vi "LJUD_GetNextResult.vi"(6 "GetFirst":bool=TRUE, 8 "error in":errorcluster, 11 "Handle In":i32) -> (0 "error out":errorcluster, 1 "LJE_NO_MORE_DATA_AVAILABLE":bool=TRUE, 2 "Value":dbl format="%.2f", 3 "Handle Out":i32, 5 "Channel":i32, 7 "IOType":i32)   [LabVIEW 2020]
doc: "This VI implements GetFirstResult and\nGetNextResult, which are used to step\nthrough the list of results in order.\n\nThis is a traditional technique UD\nfunction ... Add-Add-Go-Get-Get.\nSee Section 4.1 of the device's\ndatasheet for more information."
uses:
  labjackud.dll
panel:
  # "This VI implements GetFirstResult and\nGetNextResult, which are used to step\nthrough the list of results in order.\n\nThis is a traditional technique UD\nfunction ... Add-Add-Go-Get-Get.\nSee Section 4.1 of the device's\ndatasheet for more information."
  # "This VI is used for GetFirst or GetNext."
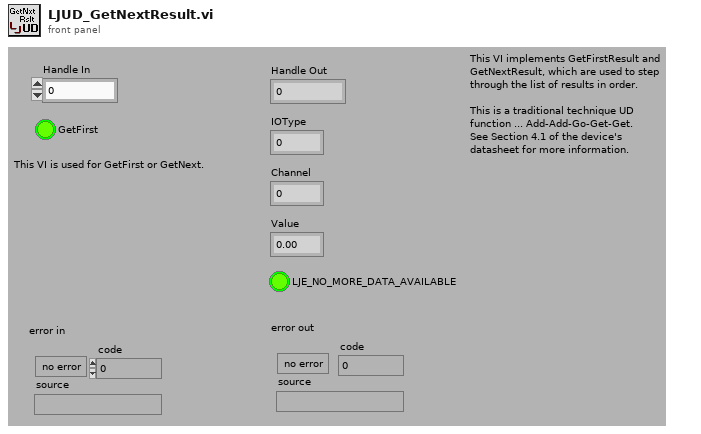
[diagram p1: front panel]
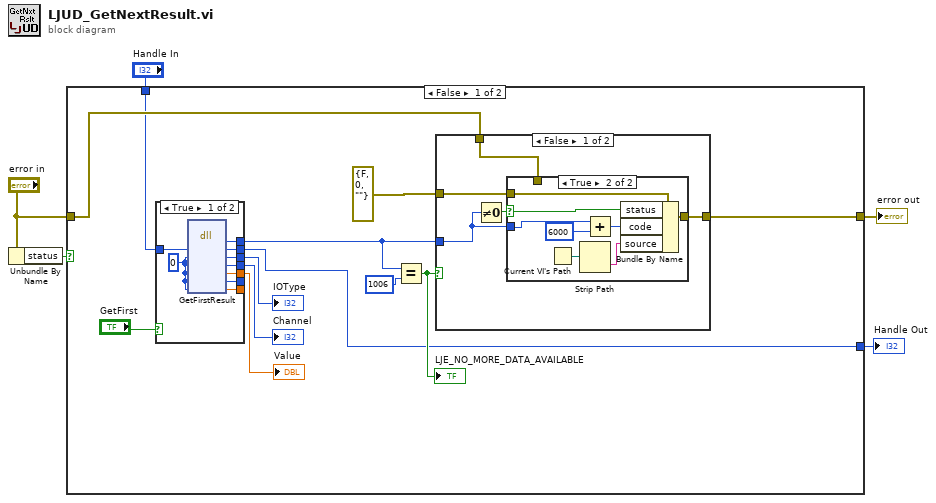
[diagram p0: block diagram]
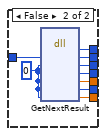
[diagram p4: hidden frame]
diagram:
  n1 = Unbundle By Name("error in") -> ("status"=w4:bool)
  n2 = case shown="False" w4 {
    tunnel: [w9 w52] -> w5
    tunnel: "error in" -> [w8 w52]
    tunnel: "Handle In" -> [w7 w51]
    tunnel: [w6 w51] -> w1
    frame False {
      n3 = case shown="True" "GetFirst" {
        tunnel: w7 -> [w41 w50]
        tunnel: [w40 w49] -> w17
        tunnel: [w39 w48] -> w13
        tunnel: [w38 w47] -> w6
        tunnel: [w36 w45] -> w15
        tunnel: [w35 w44] -> w14
        tunnel: [w34 w43] -> _
        tunnel: [w33 w42] -> _
        frame True {
          w37 = 0 ("IOType")
          n4 = dll-call lib="labjackud.dll" fn="GetFirstResult"("Handle"=w41, "IOType"=w37, "Channel"=w37, "Value"=w37, "x1"=w37, "UserData"=w37) -> (w39:i32, "Handle"=w38:i32, "IOType"=w36:i32, "Channel"=w35:i32, "Value"=w40:dbl, "x1"=w34:i32, "UserData"=w33:dbl)  [unwired: 3 in, 2 out]
        }
        frame False {
          w46 = 0 ("IOType")
          n5 = dll-call lib="labjackud.dll" fn="GetNextResult"("Handle"=w50, "IOType"=w46, "Channel"=w46, "Value"=w46, "x1"=w46, "UserData"=w46) -> (w48:i32, "Handle"=w47:i32, "IOType"=w45:i32, "Channel"=w44:i32, "Value"=w49:dbl, "x1"=w43:i32, "UserData"=w42:dbl)  [unwired: 3 in, 2 out]
        }
      }
      "IOType" <- w15
      "Channel" <- w14
      "Value" <- w17
      n6 = Equal?(x=w13, y=1006) -> (x = y?=w11:bool)
      "LJE_NO_MORE_DATA_AVAILABLE" <- w11
      n7 = case shown="False" w11 {
        tunnel: w13 -> [w21 _]
        tunnel: errorcluster {"status"=FALSE, "code"=0, "source"=""} ("error IO") -> [w20 _]
        tunnel: [w19 w32] -> w9
        tunnel: w8 -> [w18 w32]
        frame False {
          n8 = Not Equal To 0?(x=w21) -> (x != 0?=w22:bool)
          n9 = case shown="True" w22 {
            selector: w22 -> [_ w30]
            tunnel: [w23 w31] -> w19
            tunnel: w20 -> [_ w29]
            tunnel: w21 -> [_ w25]
            tunnel: w18 -> [w23 _]
            frame False {
            }
            frame True {
              n10 = Current VI's Path() -> (path=w27:path)
              n11 = Strip Path(path=w27) -> (name=w28:string)  [unwired: 1 out]
              n12 = Add(x=w25, y=6000) -> (x+y=w26:i32)
              n13 = Bundle By Name(cluster=w29, "status"=w30, "code"=w26, "source"=w28) -> (w31:errorcluster)
            }
          }
        }
        frame True {
        }
      }
    }
    frame True {
    }
  }
  "error out" <- w5
  "Handle Out" <- w1
